vi "DatabaseHand_Group_GetAll.vi"(8 "error in (no error)":errorcluster, 11 "Database RefNum in":T1) -> (0 "error out":errorcluster, 1 "database string string":string, 2 "database array":string[][](array[string]), 3 "Database RefNum out":T1)   [LabVIEW 2016]
doc: "This VI finds the RefNum of an existing object with the input Name or creates a new object if the Name is not found or Name is unwired or an empty string.\nCopyright 2001 VI Engineering, Inc."
uses:
  DatabaseHand_RefNum.ctl
  DatabaseHand_Function.ctl
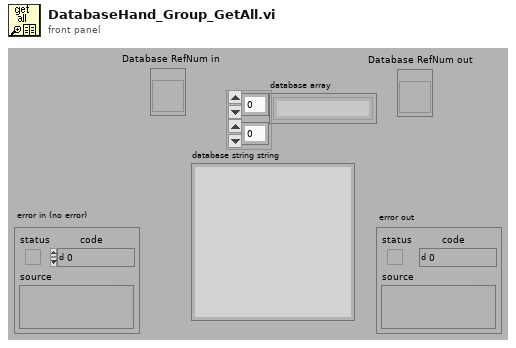
[diagram p1: front panel]
types:
  T1 = typedef "DatabaseHand_RefNum.ctl" = refnum<vi>
  T2 = typedef "DatabaseHand_Function.ctl" = enum16{"Reset", "Register", "Get Data", "Set Data", "Unregister", "Test", "Get Objects", "Delete Data"}
  T3 = typedef "Database_Refnum.ctl" = refnum<vi>
  T4 = typedef "DatabaseHand_Element.ctl" = cluster{"name":string, "Database":T5[]}
  T5 = typedef "DatabaseHan_DatabaseElement.ctl" = cluster{"name":string, "value":string, "type":string, "unit":string, "permissions":string, "enqueued":bool, "group":string}
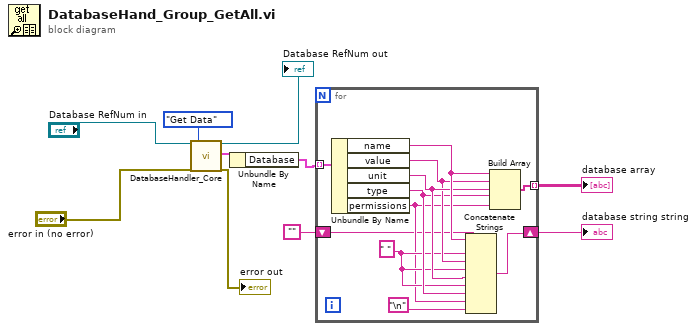
[diagram p0: block diagram]
diagram:
  n1 = call "DatabaseHandler_Core.vi"("Object Refnum In"="Database RefNum in", "error in (no error)"="error in (no error)", "Function (Get Data)"=DatabaseHand_Function."Get Data") -> ("Object Refnum out"=→"Database RefNum out":T3, "Object Data Out"=w4:T4, "error out"=→"error out":errorcluster)  [unwired: 4 in, 10 out]
  n2 = Unbundle By Name(w4) -> ("Database"=w3:T5[])
  n3 = for {
    tunnel: w3 -> [w21] mode=indexing
    tunnel: [w20] -> w10 mode=indexing
    shift-right: [w12] -> w8
    shift-left: "" -> [w11]
    w15 = " "
    n4 = Unbundle By Name(w21) -> ("name"=w19:string, "value"=w17:string, "unit"=w18:string, "type"=w16:string, "permissions"=w14:string)
    n5 = Concatenate Strings(w11, w19, w15, w17, w15, w18, w15, w16, w14, "\n") -> (w12:string)
    n6 = Build Array(w19, w17, w18, w16, w14) -> (w20:string[])
  }
  "database array" <- w10
  "database string string" <- w8
